vi "Logic Threshold to Byte.vi"(11 "Logic Threshold (%)":dbl) -> (3 "Threshold Byte":u8 format="%08b")   [LabVIEW 2014, in "SLSC configuration Shared.lvlib"]
uses:
  SLSC configuration Shared.lvlib
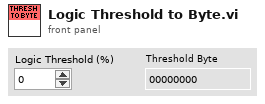
[diagram p1: front panel]
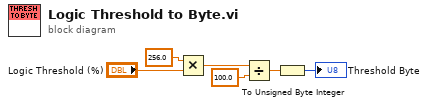
[diagram p0: block diagram]
diagram:
  n1 = Multiply(x=256.0, y="Logic Threshold (%)") -> (x*y=w4:dbl)
  n2 = Divide(x=w4, y=100.0) -> (x/y=w6:dbl)
  n3 = To Unsigned Byte Integer(number=w6) -> (unsigned 8bit integer=→"Threshold Byte":u8)
